vi "Autonomous Independent.vi"   [LabVIEW 2012]
doc: "This VI is called when autonomous begins, and will automatically be terminated when autonomous ends. You can carry out timed or sensor driven robot movement independently without needing to return to the caller."
uses:
  Robot Global Data.vi
  System Set Points and States.vi
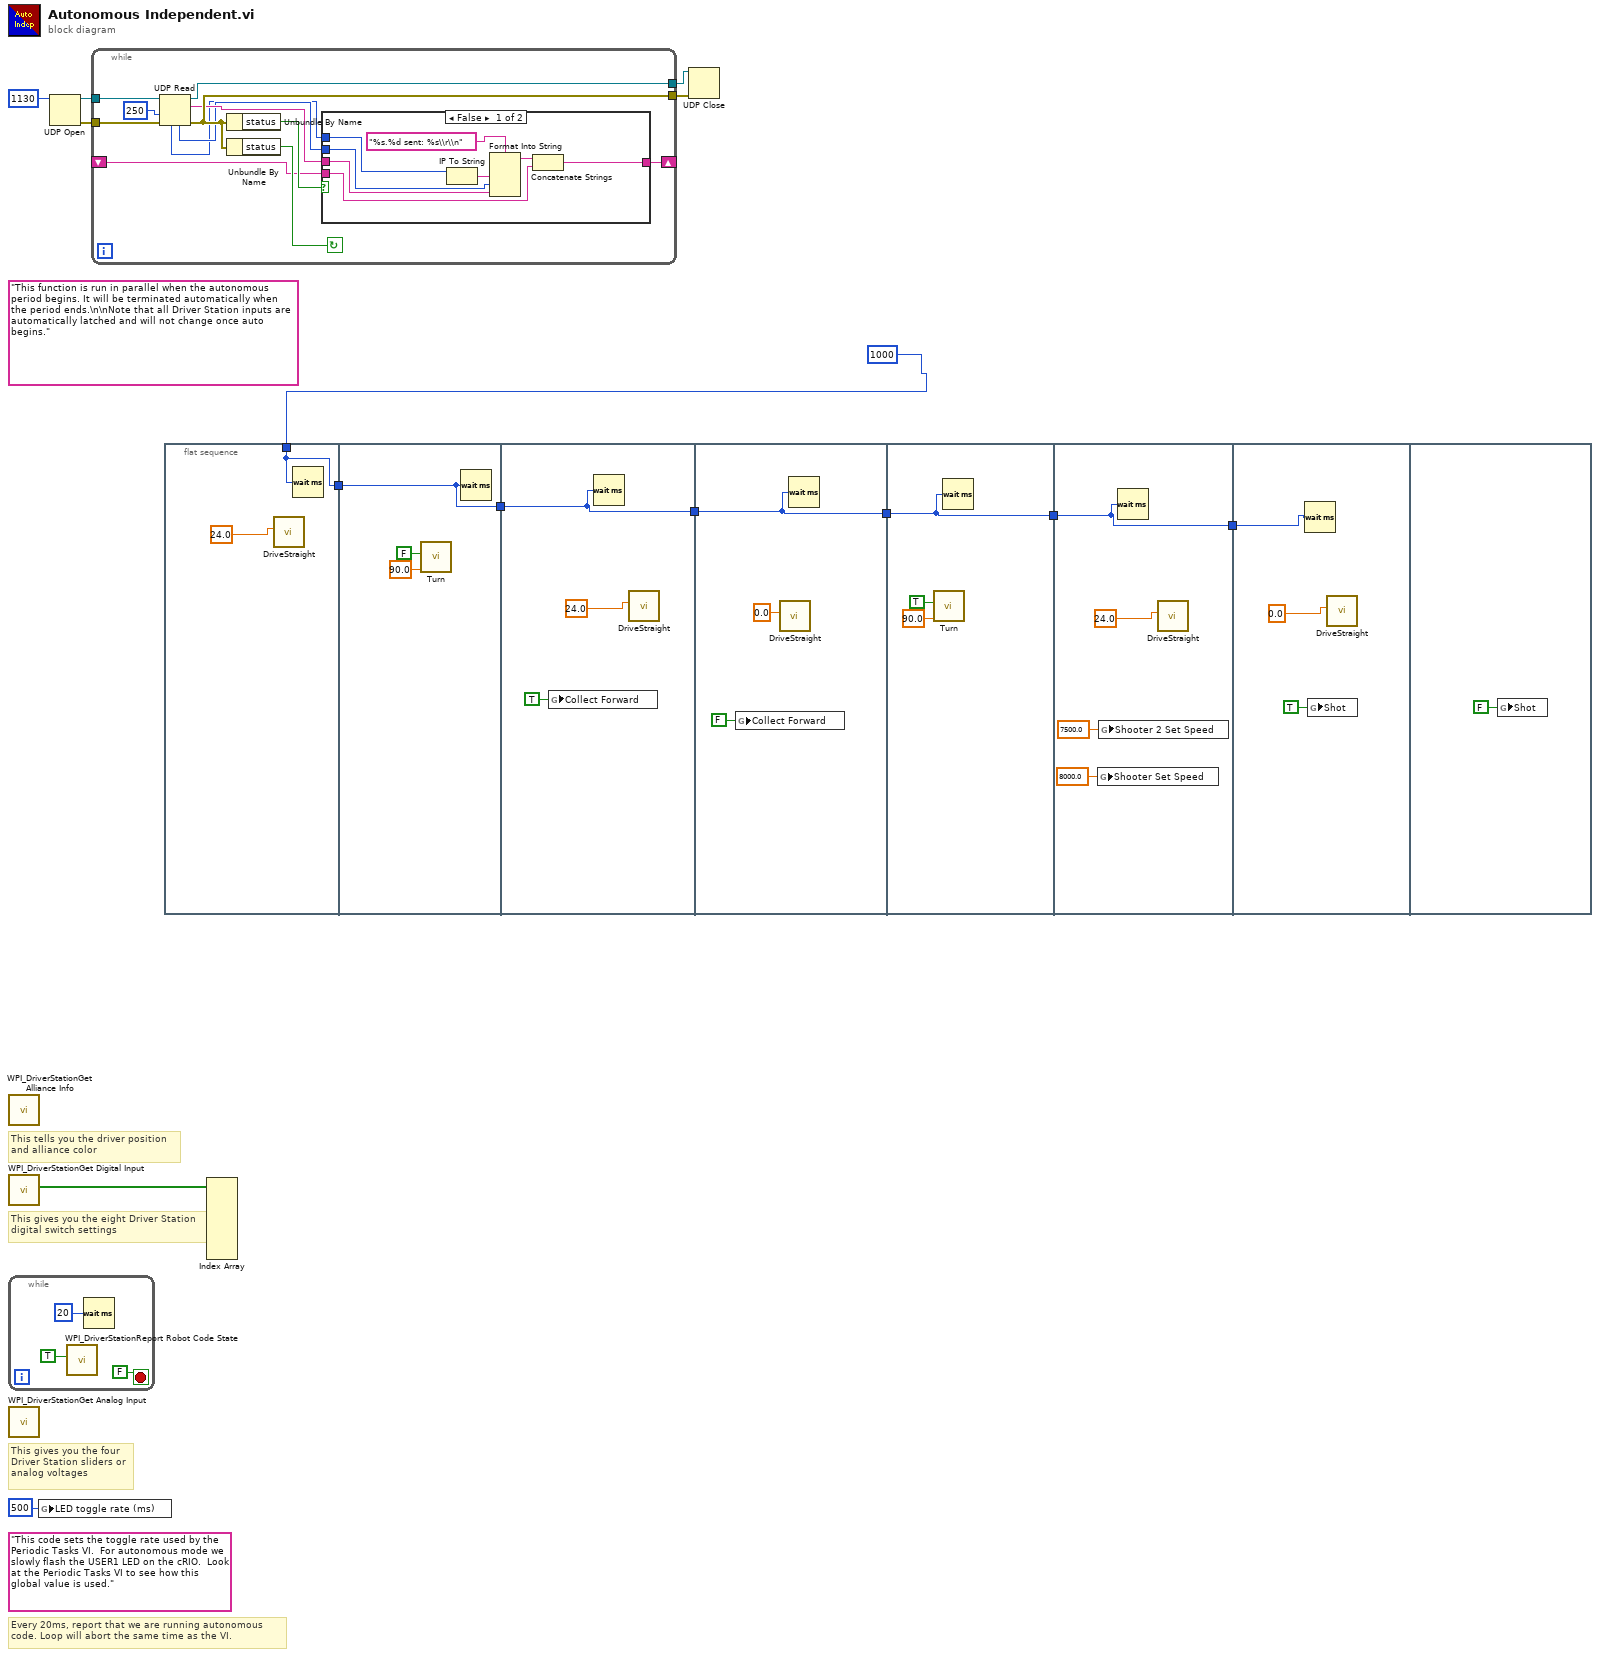
[diagram p0: block diagram]
diagram:
  (unwired) "This code sets the toggle rate used by the Periodic Tasks VI.  For autonomous mode we slowly flash the USER1 LED on the cRIO.  Look at the Periodic Tasks VI to see how this global value is used."
  (unwired) "This function is run in parallel when the autonomous period begins. It will be terminated automatically when the period ends.\n\nNote that all Driver Station inputs are automatically latched and will not change once auto begins."
  # "Every 20ms, report that we are running autonomous\ncode. Loop will abort the same time as the VI."
  # "This tells you the driver position\nand alliance color"
  # "This gives you the eight Driver Station\ndigital switch settings"
  # "This gives you the four\nDriver Station sliders or\nanalog voltages"
  n1 = call <vilib>:"WPI_DriverStationGet Alliance Info.vi"() -> ()  [unwired: 12 out]
  n2 = call <vilib>:"WPI_DriverStationGet Digital Input.vi"() -> ("Driver Station Digital Input (1-8)"=w9:bool[])  [unwired: 11 out]
  n3 = while {
    stop <- FALSE stop-if-true
    n4 = call <vilib>:"WPI_DriverStationReport Robot Code State.vi"("Autonomous"=TRUE) -> ()  [unwired: 10 in, 1 out]
    n5 = Wait (ms)(milliseconds to wait=u32 20) -> ()  [unwired: 1 out]
  }
  n6 = call <vilib>:"WPI_DriverStationGet Analog Input.vi"() -> ()  [unwired: 12 out]
  n7 = global write "Robot Global Data.vi" "LED toggle rate (ms)"(u32 500 ("LED ms toggle rate")) -> ()
  n8 = UDP Open(11:u16 1130 ("port")) -> (port=w12:refnum<k16>, 0:w14:errorcluster)  [unwired: 4 in, 1 out]
  n9 = while {
    tunnel: w14 -> [w29]
    tunnel: w12 -> [w28]
    tunnel: [w27] -> w11
    tunnel: [w24] -> w10
    shift-right: [w18] -> _
    shift-left: _ -> [w19]
    stop <- w25 continue-if-true
    n10 = UDP Read(connection ID=w28, timeout ms (25000)=250, 8:w29) -> (data out=w22:string, error out=w24:errorcluster, 3:w27:refnum<k16>, 4:w21:u16, 6:w20:u32)  [unwired: 1 in]
    n11 = Unbundle By Name(w24) -> ("status"=w23:bool)
    n12 = Unbundle By Name(w24) -> ("status"=w25:bool)
    n13 = case shown="False" w23 {
      tunnel: w22 -> [w31 _]
      tunnel: w21 -> [w35 _]
      tunnel: w20 -> [w33 _]
      tunnel: w19 -> [w32 w38]
      tunnel: [w30 w38] -> w18
      frame False {
        n14 = IP To String(2:w33) -> (0:w34:string)  [unwired: 1 in]
        n15 = Format Into String(format string="%s.%d sent: %s\\r\\n", w34, w35, w31) -> (resulting string=w37:string)  [unwired: 2 in, 1 out]
        n16 = Concatenate Strings(w37, w32) -> (w30:string)
      }
      frame True {
      }
    }
  }
  n17 = flat-sequence {
    tunnel: u32 1000 ("milliseconds to wait") -> [w39]
    tunnel: [w39] -> w6
    tunnel: w6 -> [w41]
    tunnel: [w41] -> w5
    tunnel: w5 -> [w44]
    tunnel: [w44] -> w4
    tunnel: w4 -> [w47]
    tunnel: [w47] -> w3
    tunnel: w3 -> [w50]
    tunnel: [w50] -> w2
    tunnel: w2 -> [w53]
    tunnel: [w53] -> w1
    tunnel: w1 -> [w58]
    frame #0 {
      n18 = call "DriveStraight.vi"("Drive Distance (in)"=24.0 ("Drive Dist")) -> ()  [unwired: 11 in]
      n19 = Wait (ms)(milliseconds to wait=w39) -> ()  [unwired: 1 out]
    }
    frame #1 {
      n20 = call "Turn.vi"("Gyro Setpoint"=90.0, "Turn Right?"=FALSE) -> ()  [unwired: 10 in]
      n21 = Wait (ms)(milliseconds to wait=w41) -> ()  [unwired: 1 out]
    }
    frame #2 {
      n22 = global write "System Set Points and States.vi" "Collect Forward"(TRUE ("Collect Forward")) -> ()
      n23 = Wait (ms)(milliseconds to wait=w44) -> ()  [unwired: 1 out]
      n24 = call "DriveStraight.vi"("Drive Distance (in)"=24.0 ("Drive Dist")) -> ()  [unwired: 11 in]
    }
    frame #3 {
      n25 = global write "System Set Points and States.vi" "Collect Forward"(FALSE ("Collect Forward")) -> ()
      n26 = call "DriveStraight.vi"("Drive Distance (in)"=0.0) -> ()  [unwired: 11 in]
      n27 = Wait (ms)(milliseconds to wait=w47) -> ()  [unwired: 1 out]
    }
    frame #4 {
      n28 = call "Turn.vi"("Gyro Setpoint"=90.0, "Turn Right?"=TRUE) -> ()  [unwired: 10 in]
      n29 = Wait (ms)(milliseconds to wait=w50) -> ()  [unwired: 1 out]
    }
    frame #5 {
      n30 = global write "System Set Points and States.vi" "Shooter Set Speed"(8000.0 ("Shooter Set Speed")) -> ()
      n31 = global write "System Set Points and States.vi" "Shooter 2 Set Speed"(7500.0 ("Shooter 2 Set Speed")) -> ()
      n32 = Wait (ms)(milliseconds to wait=w53) -> ()  [unwired: 1 out]
      n33 = call "DriveStraight.vi"("Drive Distance (in)"=24.0 ("Drive Dist")) -> ()  [unwired: 11 in]
    }
    frame #6 {
      n34 = Wait (ms)(milliseconds to wait=w58) -> ()  [unwired: 1 out]
      n35 = global write "System Set Points and States.vi" "Shot"(TRUE ("Shot")) -> ()
      n36 = call "DriveStraight.vi"("Drive Distance (in)"=0.0 ("Drive Dist")) -> ()  [unwired: 11 in]
    }
    frame #7 {
      n37 = global write "System Set Points and States.vi" "Shot"(FALSE ("Shot")) -> ()
    }
  }
  n38 = Index Array(array=w9) -> ()  [unwired: 8 in, 8 out]
  n39 = UDP Close(connection ID=w11, 8:w10) -> ()  [unwired: 2 out]
